vi "Tool Q LEIN stroke Start Pressure Monitoring.vi"(1 "Retry on err (F)":bool, 7 "Input value":dbl, 11 "error in (no error)":errorcluster) -> (4 "LEIN custom reply Q":T1, 15 "error out":errorcluster)   [LabVIEW 2011]
uses:
  LEINmaster/Defenitions/LEIN custom reply Q.ctl
  LEINmaster/Defenitions/LEIN Reply Holder.ctl
  LEINmaster/Defenitions/LEIN CMD Cluster.ctl
  LEINmaster/Defenitions/LEIN CMD List.ctl
  LEINmaster/Defenitions/LEIN Structure variations.ctl
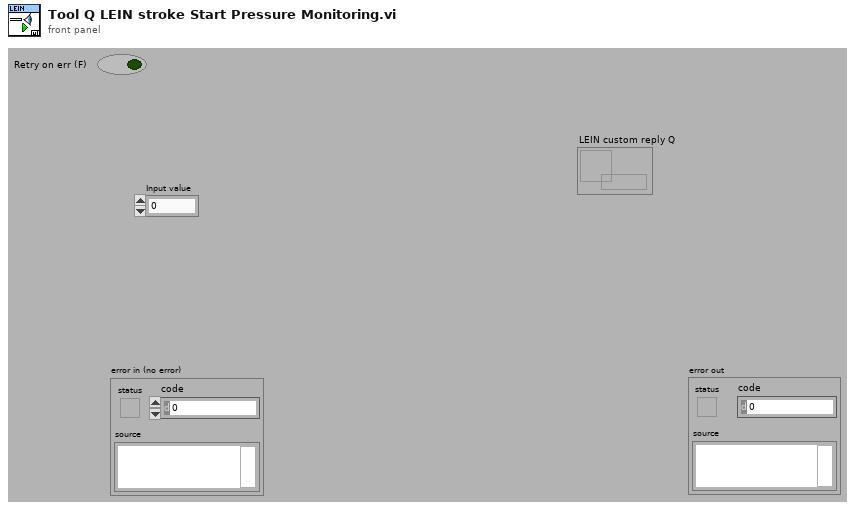
[diagram p1: front panel]
types:
  T1 = typedef "LEIN custom reply Q.ctl" = refnum<queue>
  T2 = enum16{"big-endian, network order", "native, host order", "little-endian"}
  T3 = typedef "LEIN Structure variations.ctl" = enum16{"LEIN08", "LEIN31", "LEIN63"}
  T4 = typedef "LEIN CMD Cluster.ctl" = cluster{"SID":u8, "ANF":bool, "CMD":T5, "DATA":u8[]}
  T5 = typedef "LEIN CMD List.ctl" = enum8{"ACTI", "TASK", "RES0", "STAT", "RES1", "RES2", "RES3", "USER"}
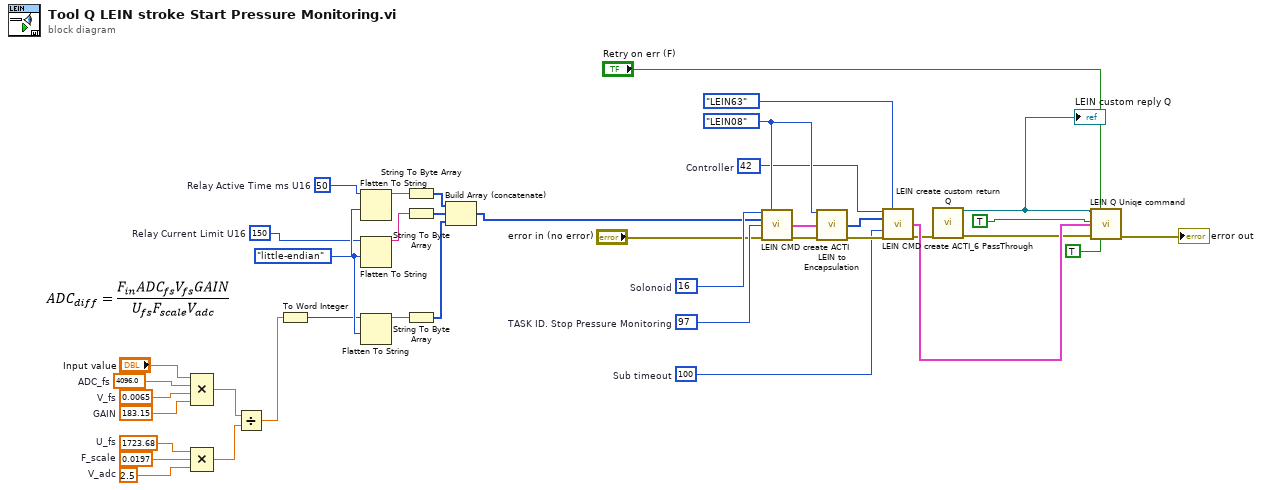
[diagram p0: block diagram]
diagram:
  w5 = 2.5  # V_adc
  w4 = 1723.68  # U_fs
  w7 = 183.15  # GAIN
  w9 = 4096.0  # ADC_fs
  w8 = 0.0065  # V_fs
  w6 = 0.0197  # F_scale
  w17 = T2."little-endian" ("byte order (0:big-endian, network order)")
  w13 = u16 150  # Relay Current Limit U16
  w14 = u16 50  # Relay Active Time ms U16
  w30 = u8 42  # Controller
  w31 = u8 16  # Solonoid
  w36 = u16 100  # Sub timeout
  w33 = u8 97  # TASK ID. Stop Pressure Monitoring
  w32 = LEIN_Structure_variations."LEIN08" ("LEIN Variation")
  n1 = Compound Arithmetic op=MULTIPLY("Input value", w9, w8, w7) -> (w3:dbl)
  n2 = Compound Arithmetic op=MULTIPLY(w4, w6, w5) -> (w2:dbl)
  n3 = Divide(x=w3, y=w2) -> (x/y=w1:dbl)
  n4 = To Word Integer(number=w1) -> (16bit integer=w11:i16)
  n5 = Flatten To String(anything=w14, byte order (0:big-endian, network order)=w17) -> (data string=w21:string)  [unwired: 2 in, 2 out]
  n6 = Flatten To String(anything=w13, byte order (0:big-endian, network order)=w17) -> (data string=w19:string)  [unwired: 2 in, 2 out]
  n7 = Flatten To String(anything=w11, byte order (0:big-endian, network order)=w17) -> (data string=w16:string)  [unwired: 2 in, 2 out]
  n8 = String To Byte Array(string=w21) -> (unsigned byte array=w20:u8[])
  n9 = String To Byte Array(string=w19) -> (unsigned byte array=w18:u8[])
  n10 = String To Byte Array(string=w16) -> (unsigned byte array=w15:u8[])
  n11 = Build Array (concatenate)(w20, w18, w15) -> (w12:u8[])
  n12 = call "LEIN CMD create ACTI.vi"("SID"=w31, "LEIN Variation"=w32, "Data"=w12, "ACTI ID"=w33, "error in (no error)"="error in (no error)") -> ("CMD"=w34:T4, "error out"=w35:errorcluster)  [unwired: 9 in]
  n13 = call "LEIN to Encapsulation.vi"("LEIN Variation"=w32, "CMD"=w34, "error in (no error)"=w35) -> ("Data and header"=w37:u8[], "error out"=w38:errorcluster)  [unwired: 8 in, 3 out]
  n14 = call "LEIN CMD create ACTI_6 PassThrough.vi"("SID"=w30, "LEIN Variation"=LEIN_Structure_variations."LEIN63", "LEIN ecapsulated data (header and data)"=w37, "Sub Timeout (ms)"=w36, "error in (no error)"=w38) -> ("CMD"=w26:T4, "error out"=w25:errorcluster)  [unwired: 9 in]
  n15 = call "LEIN create custom return Q.vi"("error in (no error)"=w25) -> ("LEIN custom reply Q"=w23:T1, "error out"=w24:errorcluster)  [unwired: 13 in]
  "LEIN custom reply Q" <- w23
  n16 = call "LEIN Q Uniqe command.vi"("LEIN custom reply Q"=w23, "Retry on err (F)"="Retry on err (F)", "Custom Q(F)"=TRUE, "CMD"=w26, "error in"=w24, "priority(F)"=TRUE) -> ("error out"=→"error out":errorcluster)  [unwired: 9 in]
